vi "Get_(X_Y_dX_dY)1.vi"(0 "(X,Y,dX,dY)":dbl[](array[numeric]), 1 "index":i32, 2 "multiplier":i32) -> (3 "X":dbl, 4 "Y":dbl, 5 "dX":dbl, 6 "dY":dbl)   [LabVIEW 2013]
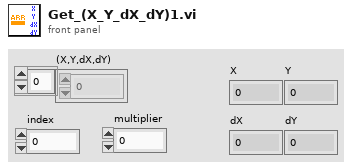
[diagram p1: front panel]
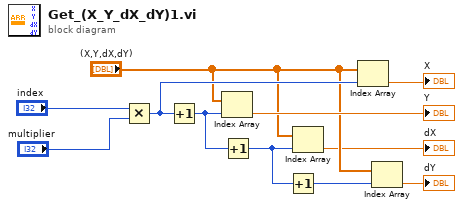
[diagram p0: block diagram]
diagram:
  n1 = Multiply(x="index", y="multiplier") -> (x*y=w8:i32)
  n2 = Increment(x=w8) -> (x+1=w7:i32)
  n3 = Index Array(array="(X,Y,dX,dY)", index=w7) -> (element=→"Y":dbl)
  n4 = Increment(x=w7) -> (x+1=w5:i32)
  n5 = Increment(x=w5) -> (x+1=w3:i32)
  n6 = Index Array(array="(X,Y,dX,dY)", index=w5) -> (element=→"dX":dbl)
  n7 = Index Array(array="(X,Y,dX,dY)", index=w8) -> (element=→"X":dbl)
  n8 = Index Array(array="(X,Y,dX,dY)", index=w3) -> (element=→"dY":dbl)
